vi "Read Query.vi"(8 "error in (no error)":errorcluster, 11 "URI-Component.Query in":refnum<class "URI-Component.Query.lvclass">) -> (0 "error out":errorcluster, 2 "Query":variant, 3 "URI-Component.Query out":refnum<class "URI-Component.Query.lvclass">)   [LabVIEW 2013, in "openURI.lvlib" / "URI-Component.Query.lvclass"]
uses:
  URI-Component.Query.lvclass
  URI-Component.Query.lvclass/URI-Component.Query.ctl
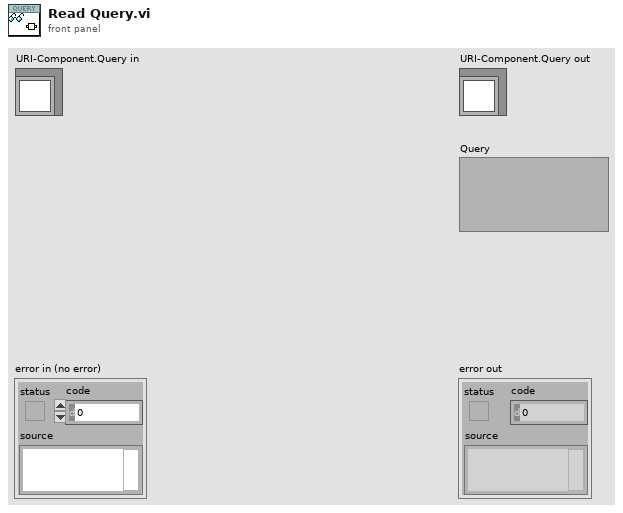
[diagram p1: front panel]
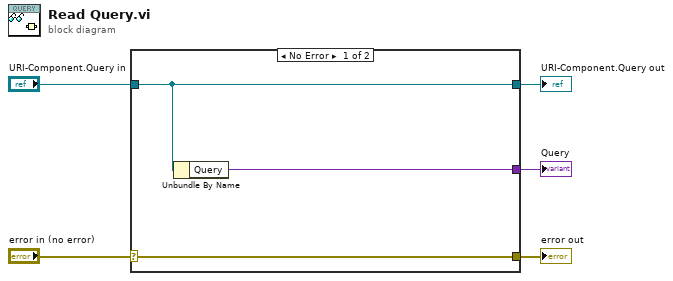
[diagram p0: block diagram]
diagram:
  n1 = case shown="No Error" "error in (no error)" {
    selector: "error in (no error)" -> [w8 w9]
    tunnel: [w8 w9] -> w4
    tunnel: [w7 w10] -> w2
    tunnel: "URI-Component.Query in" -> [w7 w10]
    tunnel: [w6 _] -> w1
    frame No Error {
      n2 = Unbundle By Name(w7) -> ("Query"=w6:variant)
    }
    frame Error {
    }
  }
  "error out" <- w4
  "URI-Component.Query out" <- w2
  "Query" <- w1
